vi "Agilent PSG MXG Series Operate N5102A Module in Output Mode.vi"() -> ()   [LabVIEW 2018]
doc: "This example shows how to operating the N5102A Module in Output Mode.\n\n<B>Note:</B>\nIt is valid only in N5172B/82B that insalls with <B>Option 003</B> or <B>Option 004</B> or <B>both</B>."
uses:
  Public/Configure/Modulation/Configure Modulation (Digital).vi
  Agilent PSG MXG Series.lvlib
panel:
  in  "Signal Type (0: I/Q)":i32(ring) items=["I/Q", "IF"]
  in  "Data Transmission Type (0: Parallel)":u16(ring) items=["Parallel", "Serial", "Parallel interleaving I/Q", "Parallel interleaving I", "Parallel interleaving Q/I"]
  in  "Logic Data Type (5: 3.3 volt CMOS signal)":u16(ring)=5 items=["Low voltage differential signal", "Low voltage TTL signal", "1.5 volt CMOS signal", "1.8 volt CMOS signal", "2.5 volt CMOS signal", "3.3 volt CMOS signal", "Simple Serial Interface"]
  in  "Multicarrier Phase (0: Fixed)":u16(ring) items=["Fixed", "Random"]
  in  "Modulation Type (6: pi/4 DQPSK)":u16(ring)=6 items=["BPSK", "QPSK", "IS-95 QPSK", "Gray Coded QPSK", "OQPSK", "IS-95 OQPSK", "pi/4 DQPSK", "8PSK", "16PSK", "D8PSK", "MSK", "2-Lvl FSK", "4-Lvl FSK", "8-Lvl FSK", "16-Lvl FSK", "C4FM", "4QAM", "16QAM", "32QAM", "64QAM", "128QAM", "256QAM", "User I/Q", "User FSK", "ASK", "UQPSK", "EDGE", "1024QAM", "VSA 16QAM", "VSA 32QAM", "VSA 64QAM", "VSA 128QAM", "VSA 256QAM", "VSA 512QAM", "VSA 1024QAM"]
  in  "VISA resource name":refnum<visa-resource-name>
  # "(c) 2016 National Instruments.  ALL RIGHTS RESERVED."
  # "This example requires the N5102A is connected to the digital bus.\nIt is valid only in N5172B/82B that insalls with Option 003 or Option 004 or both."
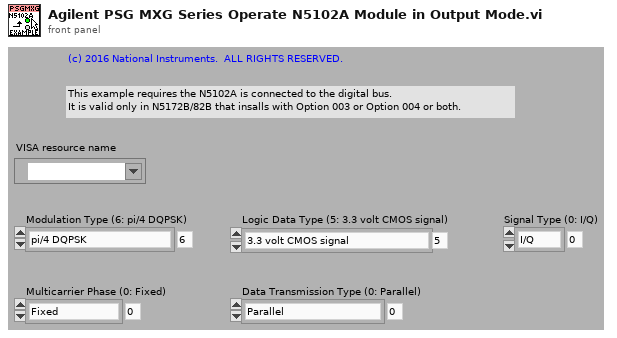
[diagram p1: front panel]
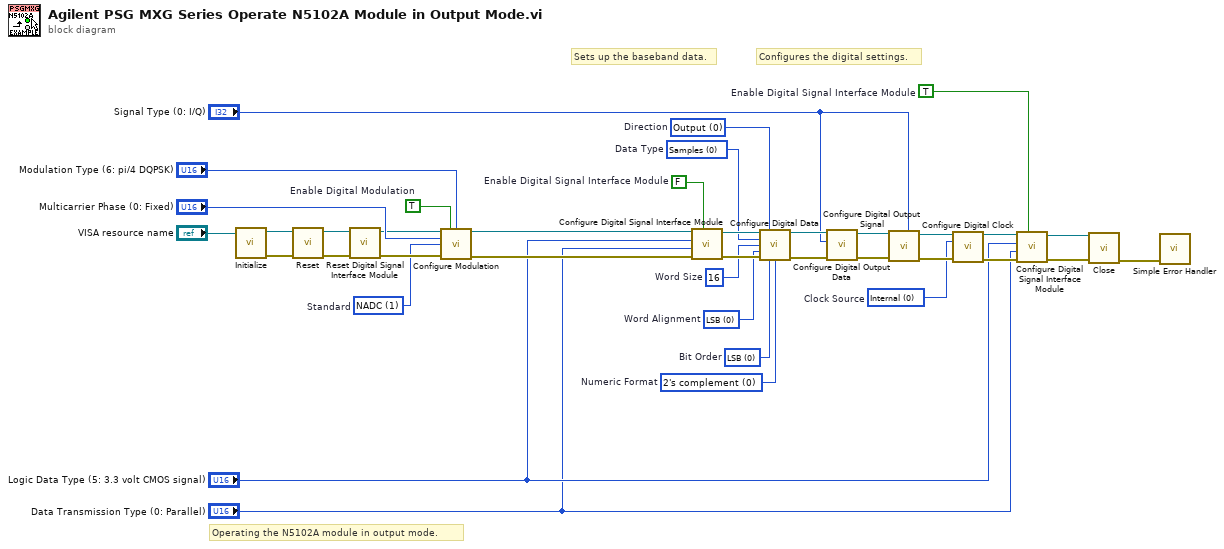
[diagram p0: block diagram]
diagram:
  w27 = u16 0 items=["Output", "Input"]  # Direction
  w15 = TRUE  # Enable Digital Signal Interface Module
  w18 = u16 0 items=["Internal", "External", "Device"]  # Clock Source
  w21 = u16 1 items=["GSM", "NADC", "PDC", "PHS", "DECT", "APCO 25 w/C4FM", "APCO w/CQPSK", "CDPD", "PWT", "EDGE", "TETRA", "Multicarrier", "Select File", "Bluetooth", "Default"]  # Standard
  w22 = u16 0 items=["2's complement", "Offset binary"]  # Numeric Format
  w23 = u16 0 items=["LSB", "MSB"]  # Bit Order
  w24 = u16 0 items=["LSB", "MSB"]  # Word Alignment
  w25 = 16  # Word Size
  w26 = u16 0 items=["Samples", "Pre-filtered Samples"]  # Data Type
  w34 = FALSE  # Enable Digital Signal Interface Module
  w37 = TRUE  # Enable Digital Modulation
  # "Configures the digital settings."
  # "Sets up the baseband data."
  # "Operating the N5102A module in output mode."
  n1 = call "Initialize.vi"("VISA resource name"="VISA resource name") -> ("error out"=w3:errorcluster, "VISA resource name out"=w4:refnum<visa-resource-name>)  [unwired: 3 in, 6 out]
  n2 = call "Reset.vi"("error in (no error)"=w3, "VISA resource name"=w4) -> ("error out"=w1:errorcluster, "VISA resource name out"=w2:refnum<visa-resource-name>)  [unwired: 8 in]
  n3 = call "Reset Digital Signal Interface Module.vi"("error in (no error)"=w1, "VISA resource name"=w2) -> ("error out"=w32:errorcluster, "VISA resource name out"=w33:refnum<visa-resource-name>)  [unwired: 8 in]
  n4 = call-poly "Configure Modulation.vi"("VISA resource name"=w33, "Enable Digital Modulation (T:Enable)"=w37, "Modulation Type (6: pi/4 DQPSK)"="Modulation Type (6: pi/4 DQPSK)", "Multicarrier Phase (0: Fixed)"="Multicarrier Phase (0: Fixed)", "Standard (1: NADC)"=w21, "error in (no error)"=w32) -> ("VISA resource name out"=w31:refnum<visa-resource-name>, "error out"=w30:errorcluster)  [unwired: 8 in]
  n5 = call "Configure Digital Signal Interface Module.vi"("Enable Digital Signal Interface Module (F:Disable)"=w34, "error in (no error)"=w30, "Data Transmission Type (0: Parallel)"="Data Transmission Type (0: Parallel)", "Logic Data Type (5: 3.3 volt CMOS signal)"="Logic Data Type (5: 3.3 volt CMOS signal)", "VISA resource name"=w31) -> ("error out"=w28:errorcluster, "VISA resource name out"=w29:refnum<visa-resource-name>)  [unwired: 5 in]
  n6 = call "Configure Digital Data.vi"("VISA resource name"=w29, "Direction (0: Output)"=w27, "Data Type (0: Samples)"=w26, "Word Size (16)"=w25, "Word Alignment (0: LSB)"=w24, "error in (no error)"=w28, "Bit Order (0: LSB)"=w23, "Numeric Format (0: 2's complement)"=w22) -> ("VISA resource name out"=w10:refnum<visa-resource-name>, "error out"=w8:errorcluster)  [unwired: 6 in]
  n7 = call "Configure Digital Output Data.vi"("error in (no error)"=w8, "Signal Type (0: I/Q)"="Signal Type (0: I/Q)", "VISA resource name"=w10) -> ("error out"=w7:errorcluster, "VISA resource name out"=w9:refnum<visa-resource-name>)  [unwired: 7 in]
  n8 = call "Configure Digital Output Signal.vi"("Signal Type (0: I/Q)"="Signal Type (0: I/Q)", "error in (no error)"=w7, "VISA resource name"=w9) -> ("error out"=w19:errorcluster, "VISA resource name out"=w20:refnum<visa-resource-name>)  [unwired: 7 in]
  n9 = call "Configure Digital Clock.vi"("VISA resource name"=w20, "Clock Source (0: Internal)"=w18, "error in (no error)"=w19) -> ("VISA resource name out"=w17:refnum<visa-resource-name>, "error out"=w16:errorcluster)  [unwired: 11 in]
  n10 = call "Configure Digital Signal Interface Module.vi"("Enable Digital Signal Interface Module (F:Disable)"=w15, "error in (no error)"=w16, "Data Transmission Type (0: Parallel)"="Data Transmission Type (0: Parallel)", "Logic Data Type (5: 3.3 volt CMOS signal)"="Logic Data Type (5: 3.3 volt CMOS signal)", "VISA resource name"=w17) -> ("error out"=w11:errorcluster, "VISA resource name out"=w12:refnum<visa-resource-name>)  [unwired: 5 in]
  n11 = call "Close.vi"("error in (no error)"=w11, "VISA resource name"=w12) -> ("error out"=w5:errorcluster)  [unwired: 9 in]
  n12 = call <vilib>:"Simple Error Handler.vi"("error in (no error)"=w5) -> ()  [unwired: 4 in, 5 out]
